vi "Fetch Waveform.vi"(8 "error in (no error)":errorcluster, 11 "Tektronix DPO MSO 2000 4000 in":refnum<class "Tektronix DPO MSO 2000 4000.lvclass">) -> (0 "error out":errorcluster, 2 "Waveform Data":waveform(dbl)[](graph), 3 "Tektronix DPO MSO 2000 4000 out":refnum<class "Tektronix DPO MSO 2000 4000.lvclass">)   [LabVIEW 2020, in "Tektronix DPO MSO 2000 4000.lvclass"]
uses:
  Tektronix DPO MSO 2000 4000.lvclass
  C:/Sandbox/Git_Sandbox/WiSpry Test Framework source code (LV20)/WiSpry Test Framework/Instruments/Instrument.lvclass
  Instrument.lvclass/Instrument.ctl
  <instrlib>/Tektronix DPO MSO 2000 4000 Series/Public/Data/Data_Low Level/Fetch Waveform (Waveform Data Type).vi
  Instrument.lvclass
  <instrlib>/Tektronix DPO MSO 2000 4000 Series/Tektronix DPO MSO 2000 4000 Series.lvlib
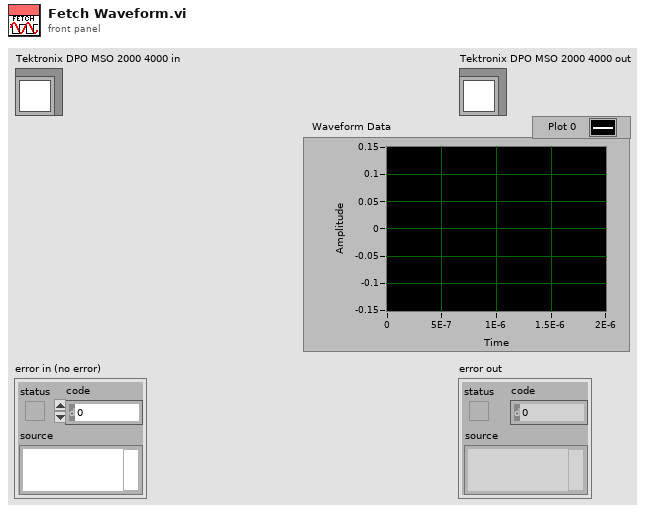
[diagram p1: front panel]
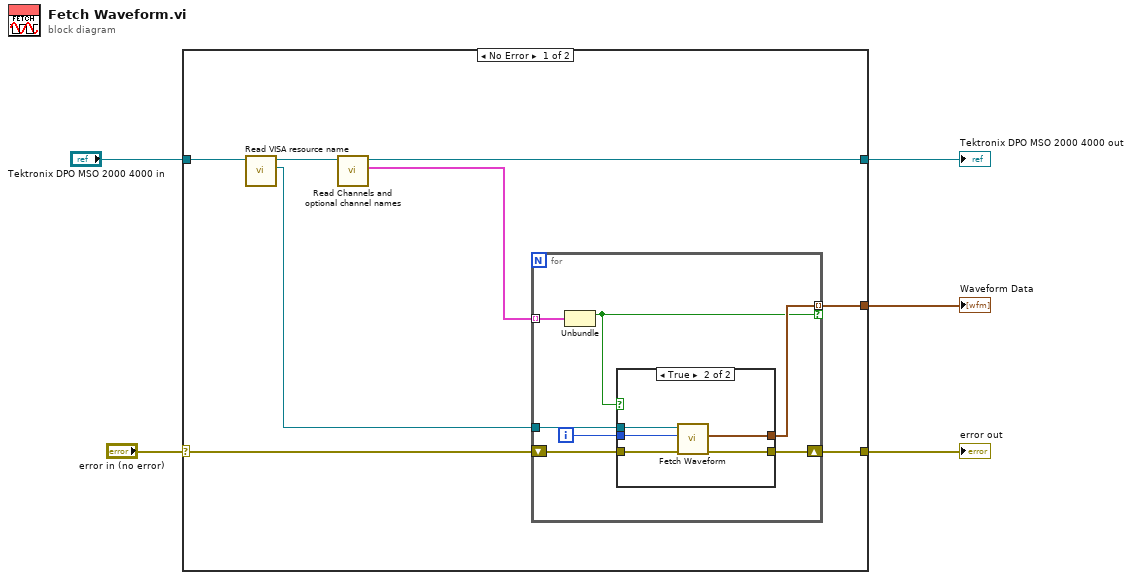
[diagram p0: block diagram]
diagram:
  n1 = case shown="No Error" "error in (no error)" {
    selector: "error in (no error)" -> [w7 w28]
    tunnel: [w8 w28] -> w1
    tunnel: [w11 w27] -> w3
    tunnel: "Tektronix DPO MSO 2000 4000 in" -> [w13 w27]
    tunnel: [w9 _] -> w2
    frame No Error {
      n2 = call "Read VISA resource name.vi"("Instrument in"=w13) -> ("VISA resource name"=w6:refnum<visa-resource-name>, "Instrument out"=w12:refnum<class "Tektronix DPO MSO 2000 4000.lvclass">)  [unwired: 9 in]
      n3 = call-dynamic "Read Channels and optional channel names.vi"("Oscilloscope in"=w12) -> ("Channels and optional channel names"=w10:cluster{"Enabled":bool, "Channel name":string}[], "Oscilloscope out"=w11:refnum<class "Tektronix DPO MSO 2000 4000.lvclass">)  [unwired: 9 in]
      n4 = for {
        tunnel: w10 -> [w20] mode=indexing
        shift-right: [w17] -> w8
        shift-left: w7 -> [w19]
        tunnel: w6 -> [w18]
        tunnel: [w16] -> w9 mode=indexing if=w15
        i -> [w14]
        n5 = Unbundle(w20) -> ("Enabled"=w15:bool)  [unwired: 1 out]
        n6 = case shown="True" w15 {
          tunnel: w19 -> [w21 w26]
          tunnel: w18 -> [_ w25]
          tunnel: [w21 w24] -> w17
          tunnel: [_ w23] -> w16
          tunnel: w14 -> [_ w22]
          frame False {
          }
          frame True {
            n7 = call-poly <instrlib>:"Fetch Waveform.vi"("error in (no error)"=w26, "Channel (0: Channel 1)"=w22, "VISA resource name"=w25) -> ("error out"=w24:errorcluster, "Waveform Data"=w23:waveform(dbl))  [unwired: 6 in, 1 out]
          }
        }
      }
    }
    frame Error {
    }
  }
  "error out" <- w1
  "Tektronix DPO MSO 2000 4000 out" <- w3
  "Waveform Data" <- w2
